vi "CalculateOctaveBands.vi"(4 "Octave":dbl, 5 "frequency range":cluster{"low band":u16, "high band":u16} {"low band" items=["16 Hz"=16, "31.5 Hz"=31, "63 Hz"=63, "125 Hz"=125, "250 Hz"=250, "500 Hz"=500, "1000 Hz"=1000, "2000 Hz"=2000, "4000 Hz"=4000, "8000 Hz"=8000, "16000 Hz"=16000]; "high band" items=["16 Hz"=16, "31.5 Hz"=31, "63 Hz"=63, "125 Hz"=125, "250 Hz"=250, "500 Hz"=500, "1000 Hz"=1000, "2000 Hz"=2000, "4000 Hz"=4000, "8000 Hz"=8000, "16000 Hz"=16000]}) -> (0 "Fmin":ext[](array[numeric]), 1 "Fmax":ext[](array[numeric]), 2 "Fctr":ext[](array[numeric]))   [LabVIEW 2014]
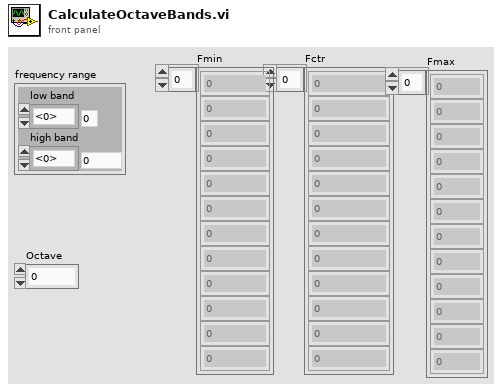
[diagram p1: front panel]
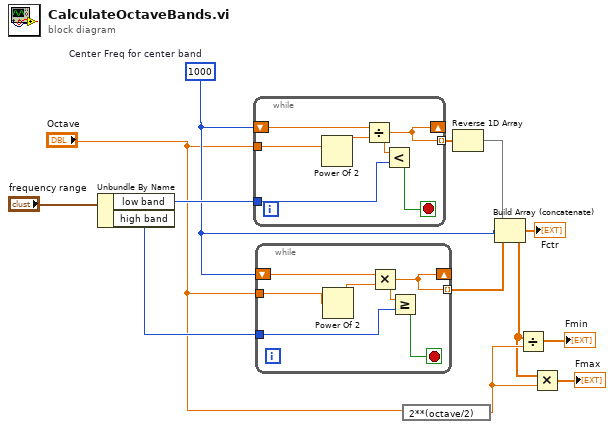
[diagram p0: block diagram]
diagram:
  w7 = 1000  # Center Freq for center band
  n1 = Unbundle By Name("frequency range") -> ("low band"=w11:u16, "high band"=w12:u16)
  n2 = while {
    tunnel: [w15] -> w6 mode=indexing
    tunnel: "Octave" -> [w13]
    shift-right: [w15] -> _
    shift-left: w7 -> [w16]
    tunnel: w11 -> [w14]
    stop <- w17 stop-if-true
    n3 = Power Of 2(x=w13) -> (2^x=w18:dbl)
    n4 = Divide(x=w16, y=w18) -> (x/y=w15:dbl)
    n5 = Less?(x=w15, y=w14) -> (x < y?=w17:bool)
  }
  n6 = while {
    tunnel: [w22] -> w8 mode=indexing
    tunnel: "Octave" -> [w20]
    shift-right: [w22] -> _
    shift-left: w7 -> [w23]
    tunnel: w12 -> [w21]
    stop <- w24 stop-if-true
    n7 = Power Of 2(x=w20) -> (2^x=w19:dbl)
    n8 = Multiply(x=w23, y=w19) -> (x*y=w22:dbl)
    n9 = Greater Or Equal?(x=w22, y=w21) -> (x >= y?=w24:bool)
  }
  n10 = expression code="2**(octave/2)"("Octave") -> (w4:dbl)
  n11 = Reverse 1D Array(array=w6) -> (reversed array=w9:dbl[])
  n12 = Build Array (concatenate)(w9, w7, w8) -> (w1:dbl[])
  "Fctr" <- w1
  n13 = Divide(x=w1, y=w4) -> (x/y=→"Fmin":dbl[])
  n14 = Multiply(x=w1, y=w4) -> (x*y=→"Fmax":dbl[])
